vi "StatusEncodeString.vi"(11 "StringIn":string) -> (2 "length":i32=24, 3 "EncodedStringOut":string)   [LabVIEW 2020]
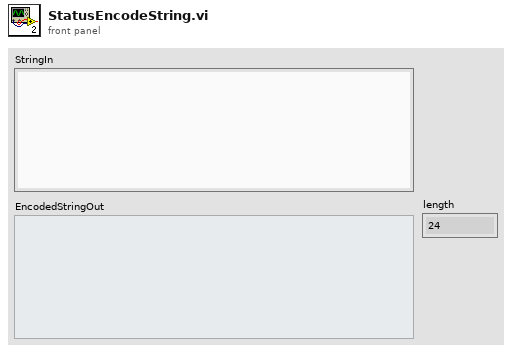
[diagram p1: front panel]
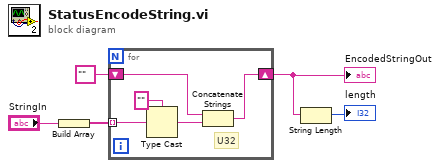
[diagram p0: block diagram]
diagram:
  n1 = Build Array("StringIn") -> (w3:string[])
  n2 = for {
    shift-right: [w10] -> w5
    shift-left: "" -> [w9]
    tunnel: w3 -> [w7] mode=indexing
    # "U32"
    n3 = Type Cast(type="", x=w7) -> (*(type *) &x=w6:string)
    n4 = Concatenate Strings(w9, w6) -> (w10:string)
  }
  "EncodedStringOut" <- w5
  n5 = String Length(string=w5) -> (length=→"length":i32)
